vi "_40_Sample_qsns_9[16].vi"() -> ()   [LabVIEW 2020]
panel:
  out "x+y":i32[](array[numeric])
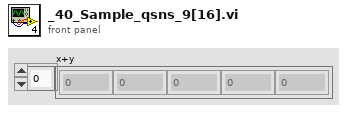
[diagram p1: front panel]
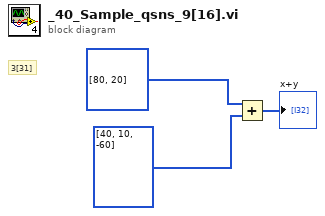
[diagram p0: block diagram]
diagram:
  # "3[31]"
  n1 = Add(x=i32[] [80, 20] ("Numeric"), y=i32[] [40, 10, -60]) -> (x+y=→"x+y":i32[])
